vi "strobe_timer.vi"() -> (0 "error out":errorcluster, 3 "notifier out":refnum<notifier>)   [LabVIEW 2013]
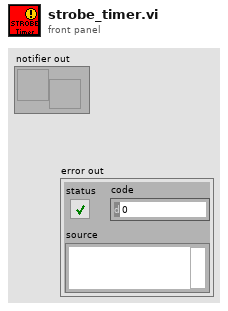
[diagram p1: front panel]
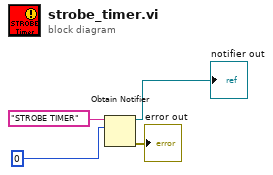
[diagram p0: block diagram]
diagram:
  n1 = Obtain Notifier(name (unnamed)="STROBE TIMER", notification data type=u32 0) -> (notifier out=→"notifier out":refnum<notifier>, error out=→"error out":errorcluster)  [unwired: 2 in, 1 out]
